vi "Tarea 3.vi"() -> ()   [LabVIEW 2019]
uses:
  Student Material/Student Material/Module 1/Exercise 3/CLD3 FGV Mode.ctl
panel:
  out "Has Time Elapsed":bool
  out "Elapsed Time (s.ss)":dbl
  in  "Time Target (s)":dbl=4.0
  in  "Timer Mode":T1
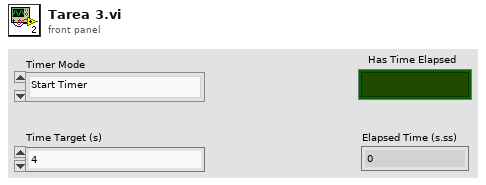
[diagram p1: front panel]
types:
  T1 = typedef "CLD3 FGV Mode.ctl" = enum16{"Start Timer", "Read Time", "Pause", "Resume"}
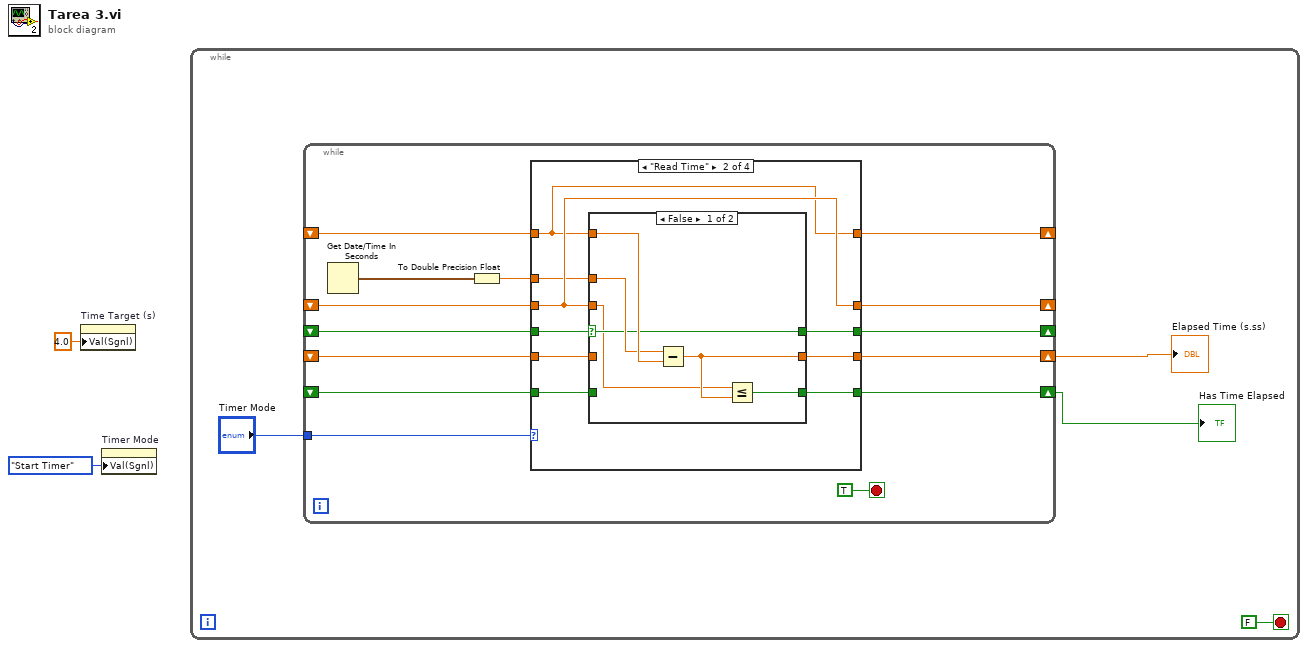
[diagram p0: block diagram]
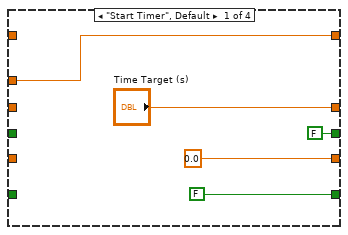
[diagram p2: hidden frame]
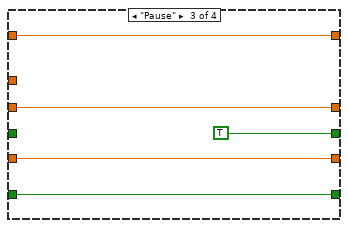
[diagram p4: hidden frame]
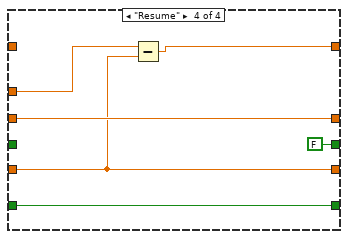
[diagram p5: hidden frame]
diagram:
  n1 = property on="Time Target (s)" class="DigNum (strict)"("Val(Sgnl)"=4.0 ("Value (Signaling)")) -> ()  [unwired: 2 in, 2 out]
  n2 = property on="Timer Mode" class="Enum (strict)"("Val(Sgnl)"=CLD3_FGV_Mode."Start Timer" ("Value (Signaling)")) -> ()  [unwired: 2 in, 2 out]
  n3 = while {
    stop <- FALSE stop-if-true
    n4 = while {
      tunnel: "Timer Mode" -> [w20]
      shift-right: [w19] -> _
      shift-left: _ -> [w16]
      shift-right: [w17] -> _
      shift-left: _ -> [w15]
      shift-right: [w7] -> w4
      shift-left: _ -> [w13]
      shift-right: [w14] -> w3
      shift-left: _ -> [w10]
      shift-right: [w9] -> _
      shift-left: _ -> [w8]
      stop <- TRUE stop-if-true
      n5 = Get Date/Time In Seconds() -> (seconds since 1Jan1904=w12:timestamp)
      n6 = To Double Precision Float(number=w12) -> (double precision float=w11:dbl)
      n7 = case shown="\"Read Time\"" w20 {
        tunnel: [w23 w31 w45 w51] -> w19
        tunnel: ["Time Target (s)" w34 w48 w54] -> w17
        tunnel: [0.0 ("Time Target (s)") w33 w47 w52] -> w7
        tunnel: w16 -> [_ w31 w45 _]
        tunnel: w15 -> [_ w34 w48 w54]
        tunnel: [FALSE w32 w46 w53] -> w14
        tunnel: w13 -> [_ w27 w47 w52]
        tunnel: w11 -> [w23 w30 _ w50]
        tunnel: w10 -> [_ w28 w46 w53]
        tunnel: [FALSE w26 TRUE FALSE] -> w9
        tunnel: w8 -> [_ w29 _ _]
        frame "Start Timer", Default {
        }
        frame "Read Time" {
          n8 = case shown="False" w29 {
            selector: w29 -> [w36 w41]
            tunnel: w34 -> [w35 _]
            tunnel: [w40 w42] -> w33
            tunnel: [w39 w43] -> w32
            tunnel: w31 -> [w38 _]
            tunnel: w30 -> [w37 _]
            tunnel: w28 -> [_ w43]
            tunnel: w27 -> [_ w42]
            tunnel: [w36 w41] -> w26
            frame False {
              n9 = Subtract(x=w37, y=w38) -> (x-y=w40:dbl)
              n10 = Less Or Equal?(x=w35, y=w40) -> (x <= y?=w39:bool)
            }
            frame True {
            }
          }
        }
        frame "Pause" {
        }
        frame "Resume" {
          n11 = Subtract(x=w50, y=w52) -> (x-y=w51:dbl)
        }
      }
    }
    "Has Time Elapsed" <- w3
    "Elapsed Time (s.ss)" <- w4
  }
